vi "Write DAQmx Task Name.vi"(8 "error in (no error)":errorcluster, 10 "DAQmx Task Name":refnum<k21>, 11 "DAQmx in":refnum<class "DAQmx.lvclass">) -> (0 "error out":errorcluster, 3 "DAQmx out":refnum<class "DAQmx.lvclass">)   [LabVIEW 2017, in "DAQmx.lvclass"]
uses:
  DAQmx.lvclass
  DAQmx.lvclass/DAQmx.ctl
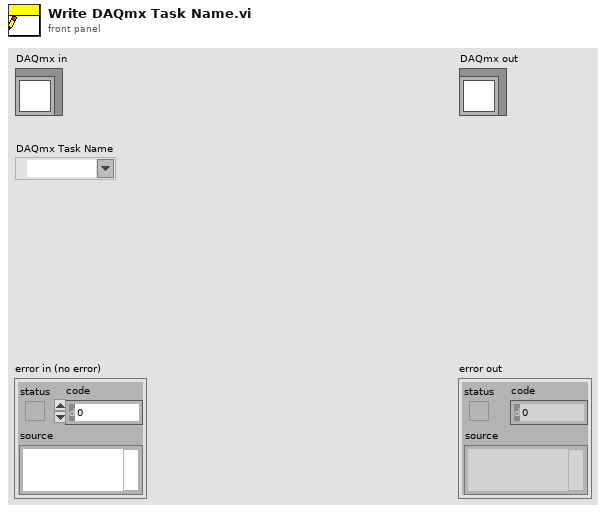
[diagram p1: front panel]
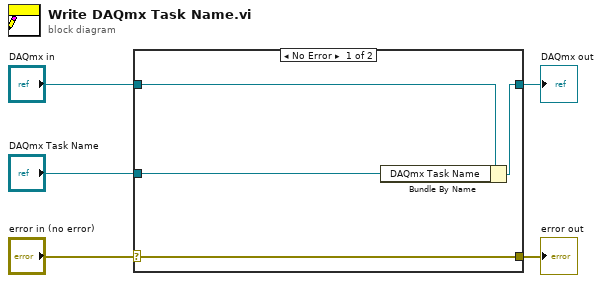
[diagram p0: block diagram]
diagram:
  n1 = case shown="No Error" "error in (no error)" {
    selector: "error in (no error)" -> [w9 w10]
    tunnel: [w9 w10] -> w4
    tunnel: [w7 w11] -> w2
    tunnel: "DAQmx in" -> [w8 w11]
    tunnel: "DAQmx Task Name" -> [w6 _]
    frame No Error {
      n2 = Bundle By Name(cluster=w8, "DAQmx Task Name"=w6) -> (w7:refnum<class "DAQmx.lvclass">)
    }
    frame Error {
    }
  }
  "error out" <- w4
  "DAQmx out" <- w2
